vi "TryAgain_theirs.vi"(4 "error in (no error)":errorcluster) -> (3 "Try again":bool)   [LabVIEW 2015]
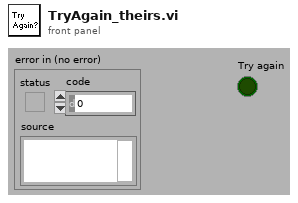
[diagram p1: front panel]
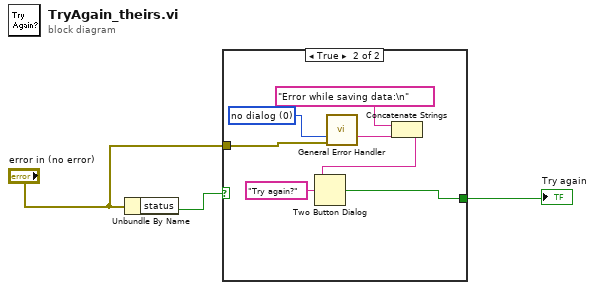
[diagram p0: block diagram]
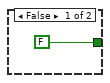
[diagram p2: hidden frame]
diagram:
  n1 = Unbundle By Name("error in (no error)") -> ("status"=w2:bool)
  n2 = case shown="True" w2 {
    tunnel: [FALSE w10] -> w3
    tunnel: "error in (no error)" -> [_ w9]
    frame False {
    }
    frame True {
      w8 = u16 0 items=["no dialog", "OK message", "continue or stop message"] ("type of dialog (OK msg:1)")
      n3 = call <vilib>:"General Error Handler.vi"("type of dialog (OK msg:1)"=w8, "error in (no error)"=w9) -> ("message"=w7:string)  [unwired: 1 in, 12 out]
      n4 = Concatenate Strings("Error while saving data:\n" ("string"), w7) -> (w6:string)
      n5 = Two Button Dialog(message=w6, 2:"Try again?" ("T button name (\"OK\")")) -> (T button?=w10:bool)  [unwired: 1 out]
    }
  }
  "Try again" <- w3
